vi "poly_error_bypass_in.vi"(9 "Error in 2":errorcluster caption="bypass error", 10 "Error in":errorcluster caption="main error") -> (1 "error out":errorcluster)   [LabVIEW 2015]
uses:
  poly_merge_errors_up.vi
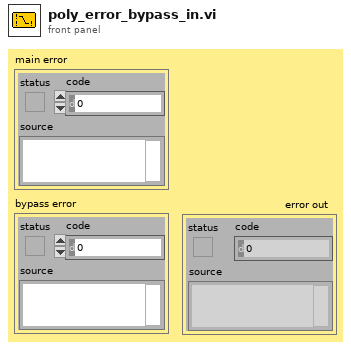
[diagram p1: front panel]
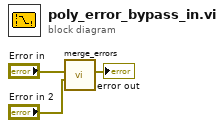
[diagram p0: block diagram]
diagram:
  n1 = call-poly "merge_errors.vi"("error in 2"="Error in 2", "error in"="Error in") -> ("error out"=→"error out":errorcluster)  [unwired: 9 in]
